vi "testSendTelServersAandB.vi"(8 "error in (no error)":errorcluster) -> (0 "error out":errorcluster)   [LabVIEW 2018]
uses:
  src/TcpServerBase/typedef/msgTypeDef.ctl
  src/TcpServerTel/typedef/queueOptionsTypeDef.ctl
  src/TcpServerTel/typedef/enqueueOptionsTypeDef.ctl
  src/FactoryTcpServer/FactoryTcpServer.lvclass
  src/TcpServer/TcpServer.lvclass/TcpServer.ctl
  src/TcpServerBase/TcpServerBase.lvclass/TcpServerBase.ctl
  src/TcpServerTel/TcpServerTel.lvclass
  home/pcortes/Documents/github/ts_labview_tcp_json/src/TcpServerBase/TcpServerBase.lvclass
  <vilib>/addons/_JKI Toolkits/Caraya/classes/Assert/Assert Equal Value_Variant.vi
  <vilib>/addons/_JKI Toolkits/Caraya/classes/Test/Test.lvclass
  src/TcpServer/TcpServer.lvclass
  src/TcpServerBase/TcpServerBase.lvclass
  <vilib>/addons/_JKI Toolkits/Caraya/classes/Assert/Assert.lvclass
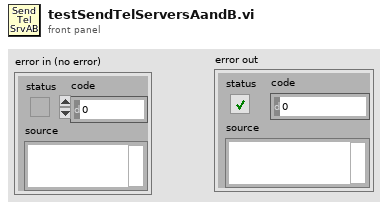
[diagram p1: front panel]
types:
  T1 = typedef "TcpServerTel.lvclass/queueOptionsTypeDef.ctl" = cluster{"EnqueueOptions":T2, "Timeout (ms)":i32}
  T2 = typedef "TcpServerTel.lvclass/enqueueOptionsTypeDef.ctl" = enum16{"lossy enqueue", "normal enqueue"}
  T3 = typedef "TcpServerBase.lvclass/msgTypeDef.ctl" = cluster{"msgName":string, "msgDetails":string}
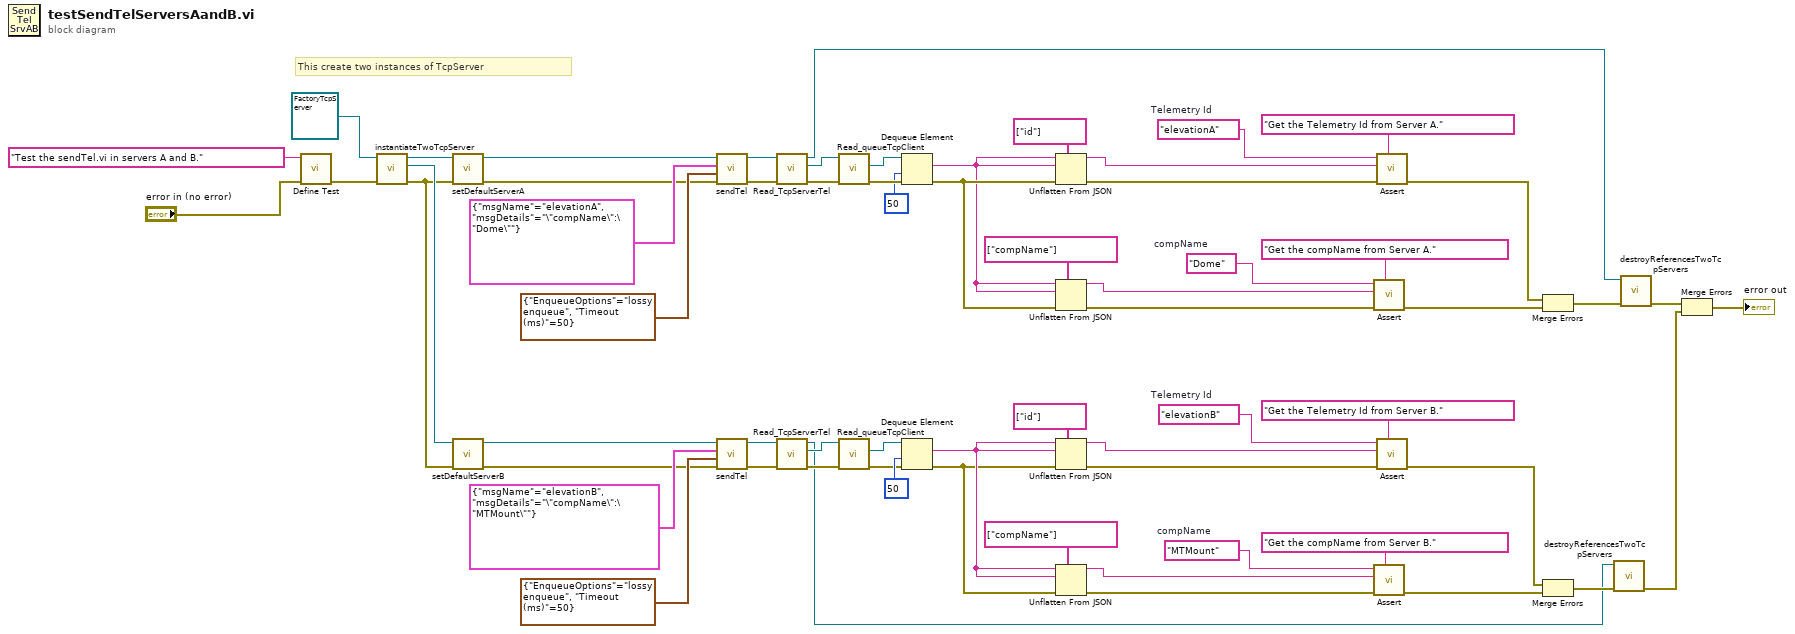
[diagram p0: block diagram]
diagram:
  w31 = "MTMount"  # compName
  w30 = "elevationB"  # Telemetry Id
  w44 = "Dome"  # compName
  w45 = "elevationA"  # Telemetry Id
  # "This create two instances of TcpServer"
  n1 = call <vilib>:"Define Test.vi"("error in (no error)"="error in (no error)", "Label (VI Title)"="Test the sendTel.vi in servers A and B.") -> ("error out"=w8:errorcluster)  [unwired: 9 in]
  n2 = call "instantiateTwoTcpServer.vi"("error in (no error)"=w8, "FactoryTcpServer in"=refnum<class "FactoryTcpServer.lvclass"> refnum) -> ("error out"=w5:errorcluster, "TcpServer 2 out"=w6:refnum<class "TcpServer.lvclass">, "TcpServer 1 out"=w7:refnum<class "TcpServer.lvclass">)  [unwired: 6 in, 1 out]
  n3 = call "setDefaultServerA.vi"("error in (no error)"=w5, "TcpServer.lvclass"=w7) -> ("error out"=w38:errorcluster, "tcpServer out"=w37:refnum<class "TcpServer.lvclass">)  [unwired: 8 in]
  n4 = call "setDefaultServerB.vi"("error in (no error)"=w5, "TcpServer.lvclass"=w6) -> ("error out"=w12:errorcluster, "tcpServer out"=w11:refnum<class "TcpServer.lvclass">)  [unwired: 8 in]
  n5 = call "sendTel.vi"("error in (no error)"=w38, "queueOptions"=T1 {"EnqueueOptions"=enum."lossy enqueue", "Timeout (ms)"=50}, "Telemetry"=T3 {"msgName"="elevationA", "msgDetails"="\"compName\":\"Dome\""} ("telData"), "tcpServer in"=w37) -> ("error out"=w54:errorcluster, "tcpServer out"=w55:refnum<class "TcpServer.lvclass">)  [unwired: 6 in]
  n6 = call "sendTel.vi"("error in (no error)"=w12, "queueOptions"=T1 {"EnqueueOptions"=enum."lossy enqueue", "Timeout (ms)"=50}, "Telemetry"=T3 {"msgName"="elevationB", "msgDetails"="\"compName\":\"MTMount\""} ("telData"), "tcpServer in"=w11) -> ("error out"=w21:errorcluster, "tcpServer out"=w20:refnum<class "TcpServer.lvclass">)  [unwired: 6 in]
  n7 = call "Read_TcpServerTel.vi"("error in (no error)"=w54, "TcpServer in"=w55) -> ("error out"=w60:errorcluster, "TcpServerTel.lvclass"=w59:refnum<class "TcpServerTel.lvclass">, "TcpServer out"=w2:refnum<class "TcpServer.lvclass">)  [unwired: 7 in]
  n8 = call "Read_TcpServerTel.vi"("error in (no error)"=w21, "TcpServer in"=w20) -> ("error out"=w15:errorcluster, "TcpServerTel.lvclass"=w16:refnum<class "TcpServerTel.lvclass">, "TcpServer out"=w1:refnum<class "TcpServer.lvclass">)  [unwired: 7 in]
  n9 = call "Read_queueTcpClient.vi"("error in (no error)"=w60, "TcpServerBase in"=w59) -> ("error out"=w58:errorcluster, "queueTcpClient"=w57:refnum<queue>)  [unwired: 7 in, 1 out]
  n10 = call "Read_queueTcpClient.vi"("error in (no error)"=w15, "TcpServerBase in"=w16) -> ("error out"=w17:errorcluster, "queueTcpClient"=w18:refnum<queue>)  [unwired: 7 in, 1 out]
  n11 = Dequeue Element(queue=w57, timeout in ms (-1)=50, error in (no error)=w58) -> (element=w52:string, error out=w53:errorcluster)  [unwired: 2 out]
  n12 = Dequeue Element(queue=w18, timeout in ms (-1)=50, error in (no error)=w17) -> (element=w23:string, error out=w22:errorcluster)  [unwired: 2 out]
  n13 = Unflatten From JSON(path=string[] ["id"], JSON string=w52, type and defaults=w52, error in (no error)=w53) -> (value=w43:string, error out=w42:errorcluster)  [unwired: 3 in]
  n14 = Unflatten From JSON(path=string[] ["compName"], JSON string=w52, type and defaults=w52, error in (no error)=w53) -> (value=w40:string, error out=w41:errorcluster)  [unwired: 3 in]
  n15 = Unflatten From JSON(path=string[] ["id"], JSON string=w23, type and defaults=w23, error in (no error)=w22) -> (value=w32:string, error out=w33:errorcluster)  [unwired: 3 in]
  n16 = Unflatten From JSON(path=string[] ["compName"], JSON string=w23, type and defaults=w23, error in (no error)=w22) -> (value=w35:string, error out=w34:errorcluster)  [unwired: 3 in]
  n17 = call-poly <vilib>:"Assert.vi"("Label"="Get the compName from Server A.", "error in (no error)"=w41, "Y"=w40, "X"=w44) -> ("error out"=w47:errorcluster)  [unwired: 7 in]
  n18 = call-poly <vilib>:"Assert.vi"("Label"="Get the compName from Server B.", "error in (no error)"=w34, "Y"=w35, "X"=w31) -> ("error out"=w28:errorcluster)  [unwired: 7 in]
  n19 = call-poly <vilib>:"Assert.vi"("Label"="Get the Telemetry Id from Server A.", "error in (no error)"=w42, "Y"=w43, "X"=w45) -> ("error out"=w46:errorcluster)  [unwired: 7 in]
  n20 = call-poly <vilib>:"Assert.vi"("Label"="Get the Telemetry Id from Server B.", "error in (no error)"=w33, "Y"=w32, "X"=w30) -> ("error out"=w29:errorcluster)  [unwired: 7 in]
  n21 = Merge Errors(w46, w47) -> (w39:errorcluster)
  n22 = Merge Errors(w29, w28) -> (w36:errorcluster)
  n23 = call "destroyReferencesTwoTcpServers.vi"("error in (no error)"=w36, "TcpServer in"=w1) -> ("error out"=w3:errorcluster)  [unwired: 8 in, 1 out]
  n24 = call "destroyReferencesTwoTcpServers.vi"("error in (no error)"=w39, "TcpServer in"=w2) -> ("error out"=w4:errorcluster)  [unwired: 8 in, 1 out]
  n25 = Merge Errors(w4, w3) -> (→"error out":errorcluster)
